vi "Multi-channel FFT(CuLab).vi"() -> ()   [LabVIEW 2020]
doc: "Computes the 1D FFT of multiple signals simultaneously using a GPU device."
uses:
  subVIs/Channel Data Type.ctl
  <vilib>/Ngene/CuLab - GPU Accelerated Toolkit/Toolkit/Low_Level/Tensor_Classes/T_Children/T2D/Controls/T2D_Dims.ctl
  <vilib>/Ngene/CuLab - GPU Accelerated Toolkit/Toolkit/Low_Level/Tensor_Classes/T_Children/T2D/Controls/T2D_Indices.ctl
  <vilib>/Ngene/CuLab - GPU Accelerated Toolkit/Toolkit/API/Array/Initialize Array/T1D/CU_Initialize Array_T1D_CSG.vi
  <vilib>/Ngene/CuLab - GPU Accelerated Toolkit/Toolkit/API/Array/Initialize Array/T2D/CU_Initialize Array_T2D_CSG.vi
  <vilib>/Ngene/CuLab - GPU Accelerated Toolkit/Toolkit/Low_Level/Tensor_Classes/T_Children/T1D/T1D_Children/T1D_CSG/Push.vi
  <vilib>/Ngene/CuLab - GPU Accelerated Toolkit/Toolkit/API/Array/Replace Array Subset (API)/CU_Replace_Array_Subset_2D_1D/CU_Replace_Array_Subset_2D_1D_CSG.vi
  <vilib>/Ngene/CuLab - GPU Accelerated Toolkit/Toolkit/API/Signal Processing/FFT/CU_FFT_Batch/T1D/CU_FFT_T1D_C2C_Batch.vi
  <vilib>/Ngene/CuLab - GPU Accelerated Toolkit/Toolkit/API/Array/Array Subset/T2D/CU_Array_Subset_T2D_CSG.vi
  <vilib>/Ngene/CuLab - GPU Accelerated Toolkit/Toolkit/API/Numeric/Absolute/T2D/CU_Absolute_T2D_CSG.vi
  <vilib>/Ngene/CuLab - GPU Accelerated Toolkit/Toolkit/API/Elementary/Exponential/Logarithm Base 10/T2D/CU_Logarithm_Base_10_T2D_SGL.vi
  <vilib>/Ngene/CuLab - GPU Accelerated Toolkit/Toolkit/API/Numeric/Multiply/T2D/CU_MultiplyC_T2D_SGL.vi
  <vilib>/Ngene/CuLab - GPU Accelerated Toolkit/Toolkit/Low_Level/Tensor_Classes/T_Children/T2D/T2D_Children/T2D_SGL/Pull.vi
  <vilib>/Ngene/CuLab - GPU Accelerated Toolkit/Toolkit/API/Array/Index Array Subset/T2D/CU_Index_Array_Subset_T2D_CSG.vi
  <vilib>/Ngene/CuLab - GPU Accelerated Toolkit/Toolkit/API/Numeric/Complex  (API)/Complex to Re Im/T1D/CU_Complex_To_Re_Im_T1D_CSG.vi
  <vilib>/Ngene/CuLab - GPU Accelerated Toolkit/Toolkit/Low_Level/Tensor_Classes/T_Children/T1D/T1D_Children/T1D_SGL/Pull.vi
  subVIs/Multi-channel FFT.lvlib
  <vilib>/ptbypt/NI_PtbyPt.lvlib
  <vilib>/Ngene/CuLab - GPU Accelerated Toolkit/Toolkit/CuLab.lvlib
  <vilib>/Ngene/CuLab - GPU Accelerated Toolkit/Toolkit/Low_Level/Tensor_Classes/T_Children/T2D/T2D_Children/T2D_SGL/T2D_SGL.lvclass
  <vilib>/Ngene/CuLab - GPU Accelerated Toolkit/Toolkit/Low_Level/Tensor_Classes/T_Children/T1D/T1D_Children/T1D_SGL/T1D_SGL.lvclass
  <vilib>/Ngene/CuLab - GPU Accelerated Toolkit/Toolkit/Low_Level/Tensor_Classes/T_Children/T1D/T1D_Children/T1D_CSG/T1D_CSG.lvclass
panel:
  in  "Execution Info":T1(tab)
  out "Current Channel":sgl[](graph)
  out "Current Spectrum":sgl[][](graph)
  in  "Channel Data":T2 items=["Pulsing Sine Wave", "Fixed Sine Wave", "Drifting Sine Wave"]
  out "GPU Exec Time":dbl format="%#_2p"
  out "Intensity Graph (dB)":sgl[][](graph)
  in  "stop":bool
  in  "Samples / channel":i32=1024
  in  "Number of channels":i32=1024
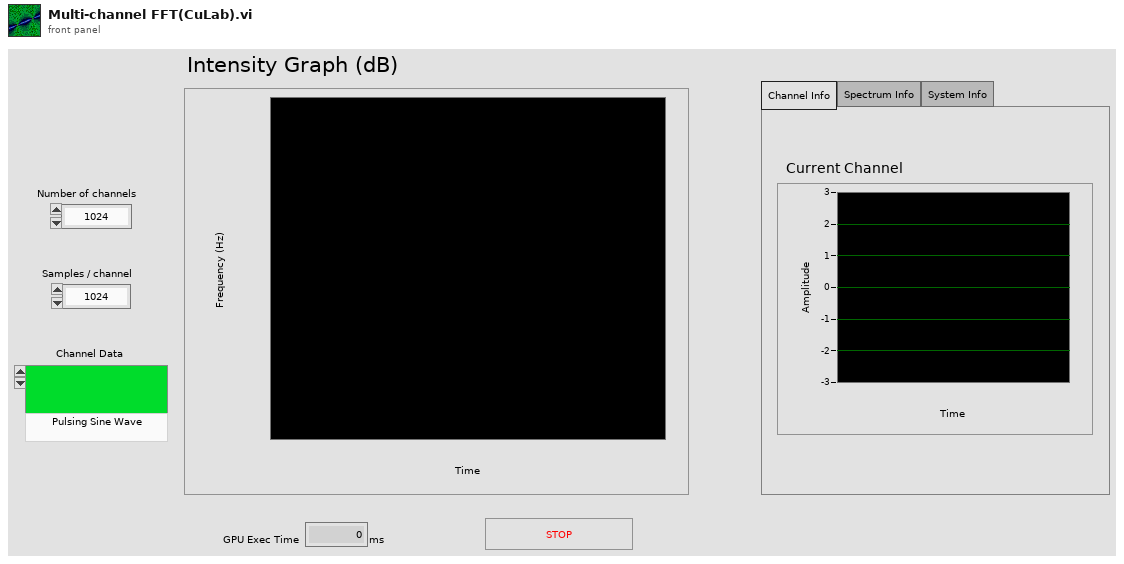
[diagram p1: front panel]
types:
  T1 = enum32{"Channel Info", "Spectrum Info", "System Info"}
  T2 = typedef "Multi-channel FFT.lvlib/Channel Data Type.ctl" = u16
  T3 = typedef "CuLab.lvlib/T2D_Dims.ctl" = cluster{"H":i32, "W":i32}
  T4 = typedef "CuLab.lvlib/T2D_Indices.ctl" = cluster{"i":i32, "j":i32}
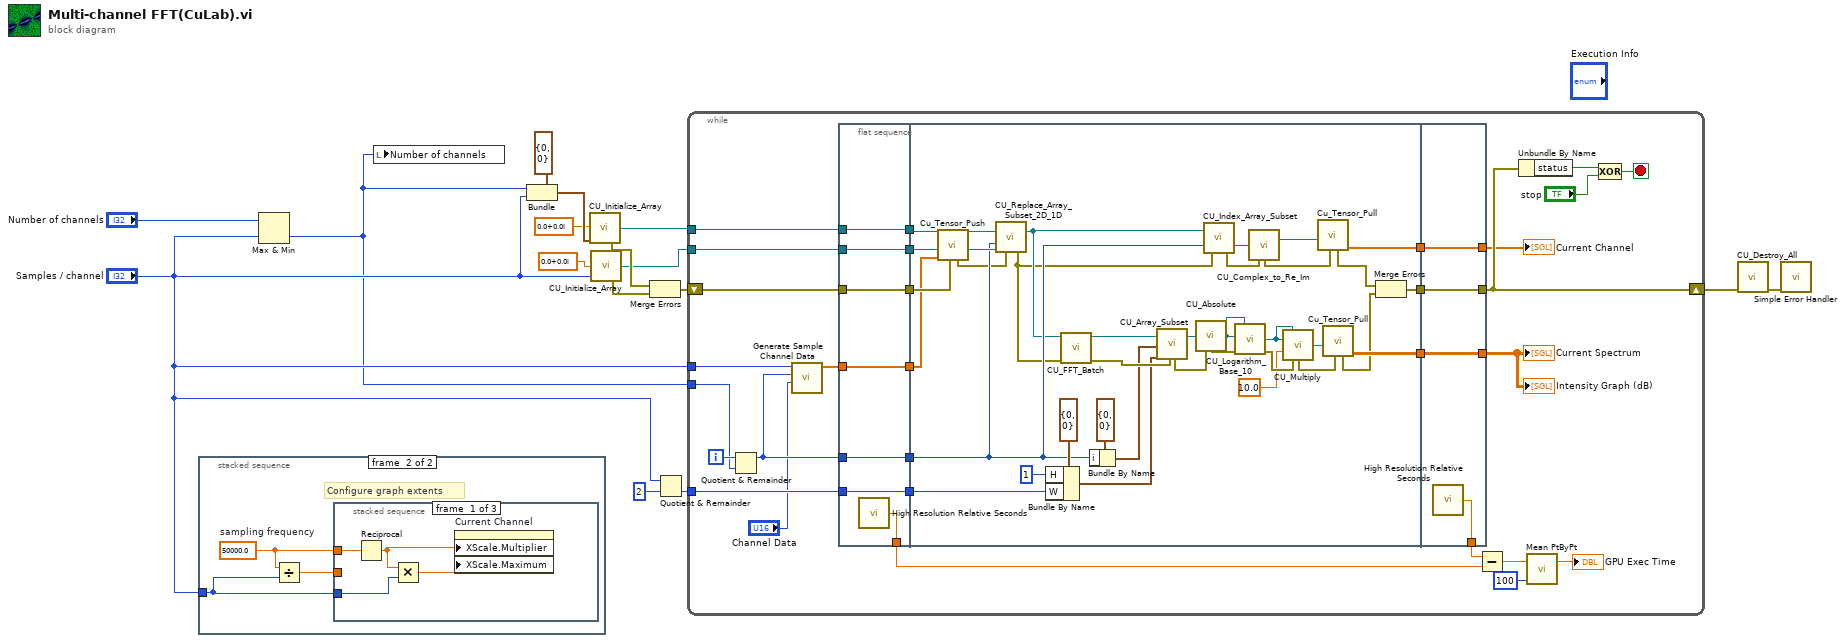
[diagram p0: block diagram]
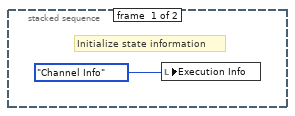
[diagram p2: hidden frame]
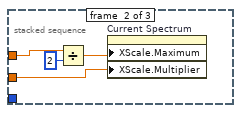
[diagram p3: hidden frame]
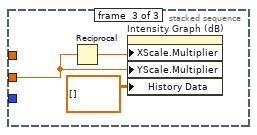
[diagram p4: hidden frame]
diagram:
  n1 = stacked-sequence {
    tunnel: "Samples / channel" -> [_ w18]
    frame #0 {
      # "Initialize state information"
      n2 = local write "Execution Info"(T1."Channel Info" ("Execution Info")) -> ()
    }
    frame #1 {
      w20 = 50000.0  # sampling frequency
      # "Configure graph extents"
      n3 = Divide(x=w20, y=w18) -> (x/y=w19:dbl)
      n4 = stacked-sequence {
        tunnel: w20 -> [w24 w27 _]
        tunnel: w19 -> [_ w28 w29]
        tunnel: w18 -> [w22 _ _]
        frame #0 {
          n5 = Reciprocal(x=w24) -> (1/x=w23:dbl)
          n6 = Multiply(x=w23, y=w22) -> (x*y=w21:dbl)
          n7 = property on="Current Channel" class="WFGraph (strict)"("XScale.Multiplier"=w23, "XScale.Maximum"=w21) -> ()  [unwired: 2 in, 2 out]
        }
        frame #1 {
          n8 = Divide(x=w27, y=2) -> (x/y=w26:dbl)
          n9 = property on="Current Spectrum" class="WFGraph (strict)"("XScale.Maximum"=w26, "XScale.Multiplier"=w28) -> ()  [unwired: 2 in, 2 out]
        }
        frame #2 {
          n10 = Reciprocal(x=w29) -> (1/x=w31:dbl)
          n11 = property on="Intensity Graph (dB)" class="IntChart (strict)"("XScale.Multiplier"=w31, "YScale.Multiplier"=w29, "History Data"=sgl[][] []) -> ()  [unwired: 2 in, 2 out]
        }
      }
    }
  }
  n12 = Max & Min(x="Number of channels", y="Samples / channel") -> (min(x,y)=w6:i32)  [unwired: 1 out]
  n13 = local write "Number of channels"(w6) -> ()
  n14 = Bundle(cluster=T3 {"H"=0, "W"=0} ("dimension sizes"), "H"=w6, "W"="Samples / channel") -> (w10:T3)
  n15 = call-poly <vilib>:"CU_Initialize_Array.vi"("element"=csg 0.0+0.0i ("CSG"), "dimension sizes"=w10) -> ("initialized Tensor"=w9:refnum<class "T2D_CSG.lvclass">, "error out"=w16:errorcluster)  [unwired: 12 in]
  n16 = call-poly <vilib>:"CU_Initialize_Array.vi"("element"=csg 0.0+0.0i ("CSG"), "dimension size"="Samples / channel") -> ("initialized Tensor"=w7:refnum<class "T1D_CSG.lvclass">, "error out"=w15:errorcluster)  [unwired: 12 in]
  n17 = Merge Errors(w16, w15) -> (w5:errorcluster)
  n18 = Quotient & Remainder(x="Samples / channel", y=2) -> (floor(x/y)=w14:i32)  [unwired: 1 out]
  n19 = while {
    shift-right: [w50] -> w2
    shift-left: w5 -> [w60]
    tunnel: w14 -> [w59]
    tunnel: "Samples / channel" -> [w53]
    tunnel: w7 -> [w33]
    tunnel: w9 -> [w61]
    tunnel: w6 -> [w32]
    i -> [w57]
    stop <- w58 stop-if-true
    n20 = Quotient & Remainder(x=w57, y=w32) -> (x-y*floor(x/y)=w52:i32)  [unwired: 1 out]
    n21 = call "Generate Sample Channel Data.vi"("channel type"="Channel Data", "channel idx"=w52, "sample size"=w53) -> ("channel data"=w56:csg[])  [unwired: 8 in]
    n22 = flat-sequence {
      tunnel: w52 -> [w64]
      tunnel: w56 -> [w65]
      tunnel: w59 -> [w66]
      tunnel: w60 -> [w67]
      tunnel: w61 -> [w68]
      tunnel: [w68] -> w46
      tunnel: [w67] -> w45
      tunnel: [w66] -> w44
      tunnel: [w65] -> w43
      tunnel: [w64] -> w42
      tunnel: [w63] -> w37
      tunnel: [w62] -> w34
      tunnel: w33 -> [w62]
      tunnel: w46 -> [w100]
      tunnel: w45 -> [w103]
      tunnel: w44 -> [w80]
      tunnel: w43 -> [w101]
      tunnel: w42 -> [w79]
      tunnel: [w76] -> w41
      tunnel: [w94] -> w40
      tunnel: [w81] -> w39
      tunnel: w34 -> [w99]
      tunnel: [w105] -> w48
      tunnel: [w106] -> w49
      tunnel: [w107] -> w50
      tunnel: w41 -> [w107]
      tunnel: w40 -> [w106]
      tunnel: w39 -> [w105]
      tunnel: [w104] -> w38
      frame #0 {
        n23 = call <vilib>:"High Resolution Relative Seconds.vi"() -> ("relative seconds"=w63:dbl)
      }
      frame #1 {
        n24 = call-poly <vilib>:"Cu_Tensor_Push.vi"("error in (no error)"=w103, "CPU_Data_1D_CSG"=w101, "T1D_CSG in"=w99) -> ("T1D_CSG out"=w98:refnum<class "T1D_CSG.lvclass">, "error out"=w77:errorcluster)  [unwired: 7 in]
        n25 = call-poly <vilib>:"CU_Replace_Array_Subset_2D_1D.vi"("Tensor in"=w100, "index"=w79, "Sub Tensor"=w98, "error in (no error)"=w77) -> ("Tensor Out"=w73:refnum<class "T2D_CSG.lvclass">, "error out"=w70:errorcluster)  [unwired: 10 in]
        n26 = Bundle By Name(cluster=T3 {"H"=0, "W"=0} ("Lengths"), "H"=1, "W"=w80) -> (w85:T3)
        n27 = call-poly <vilib>:"CU_FFT_Batch.vi"("error in"=w70, "X"=w73) -> ("error out"=w102:errorcluster, "FFT {X}"=w74:refnum<class "T2D_CSG.lvclass">)  [unwired: 8 in]
        n28 = Bundle By Name(cluster=T4 {"i"=0, "j"=0} ("Indices"), "i"=w79) -> (w83:T4)
        n29 = call-poly <vilib>:"CU_Array_Subset.vi"("Tensor in"=w74, "Indices"=w83, "Lengths"=w85, "error in (no error)"=w102) -> ("error out"=w90:errorcluster, "Dest out"=w86:refnum<class "T2D_CSG.lvclass">)  [unwired: 14 in]
        n30 = call-poly <vilib>:"CU_Absolute.vi"("x"=w86, "error in (no error)"=w90) -> ("Dest out"=w71:refnum<class "T2D_SGL.lvclass">, "error out"=w91:errorcluster)  [unwired: 12 in]
        n31 = call-poly <vilib>:"CU_Index_Array_Subset.vi"("Tensor in"=w73, "Index"=w79, "error in (no error)"=w70) -> ("error out"=w78:errorcluster, "Sub Tensor"=w95:refnum<class "T1D_CSG.lvclass">)  [unwired: 15 in]
        n32 = call-poly <vilib>:"CU_Logarithm_Base_10.vi"("Dest in"=w71, "x"=w71, "error in (no error)"=w91) -> ("log(x)"=w72:refnum<class "T2D_SGL.lvclass">, "error out"=w92:errorcluster)  [unwired: 11 in]
        n33 = call-poly <vilib>:"CU_Complex_to_Re_Im.vi"("x"=w95, "error in (no error)"=w78) -> ("Re Dest out"=w96:refnum<class "T1D_SGL.lvclass">, "error out"=w97:errorcluster)  [unwired: 11 in, 1 out]
        n34 = call-poly <vilib>:"CU_Multiply.vi"("Dest in"=w72, "x"=w72, "y"=sgl 10.0 ("single precision float"), "error in (no error)"=w92) -> ("Dest out"=w88:refnum<class "T2D_SGL.lvclass">, "error out"=w93:errorcluster)  [unwired: 10 in]
        n35 = call-poly <vilib>:"Cu_Tensor_Pull.vi"("error in (no error)"=w97, "T1D_SGL in"=w96) -> ("Dest out"=w94:sgl[], "error out"=w69:errorcluster)  [unwired: 7 in, 1 out]
        n36 = call-poly <vilib>:"Cu_Tensor_Pull.vi"("error in (no error)"=w93, "T2D_SGL in"=w88) -> ("2D_SGL_Data"=w81:sgl[][], "error out"=w75:errorcluster)  [unwired: 7 in, 1 out]
        n37 = Merge Errors(w69, w75) -> (w76:errorcluster)
      }
      frame #2 {
        n38 = call <vilib>:"High Resolution Relative Seconds.vi"() -> ("relative seconds"=w104:dbl)
      }
    }
    n39 = Subtract(x=w38, y=w37) -> (x-y=w47:dbl)
    n40 = Unbundle By Name(w50) -> ("status"=w55:bool)
    n41 = call <vilib>:"Mean PtByPt.vi"("x"=w47, "sample length"=100) -> ("mean"=→"GPU Exec Time":dbl)  [unwired: 2 in, 1 out]
    n42 = Compound Arithmetic op=XOR(w55, "stop") -> (w58:bool)
    "Current Channel" <- w49
    "Current Spectrum" <- w48
    "Intensity Graph (dB)" <- w48
  }
  n43 = call <vilib>:"CU_Destroy_All.vi"("error in"=w2) -> ("error out"=w1:errorcluster)  [unwired: 10 in]
  n44 = call <vilib>:"Simple Error Handler.vi"("error in (no error)"=w1) -> ()  [unwired: 4 in, 5 out]
